vi "fun_TimeLength2Points(ClusterOfSweepPara).vi"(10 "HDAWG Sample Rate (2.4GSa/s)":dbl=2400000000.0 format="%#_13p", 11 "AWG Sweep Parameters Time length (s)":cluster{"End":dbl, "Step":dbl, "Start":dbl}={"End"=1.5e-05, "Step"=2.0833e-08, "Start"=2e-07} caption="Sweep Parameters" {"End" min=0.0 max=40000.0 step=1.0 format="%#.3ps"; "Step" format="%.3ps"; "Start" min=0.0 max=12000000000.0 step=100000000.0 format="%#.3ps"}) -> (3 "AWG Points":cluster{"End":dbl, "Step":dbl, "Start":dbl} caption="Points" {"End" min=0.0 max=40000.0 step=1.0; "Start" min=0.0 max=12000000000.0 step=100000000.0})   [LabVIEW 2016]
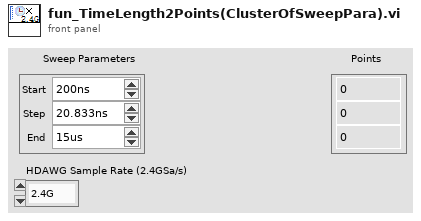
[diagram p1: front panel]
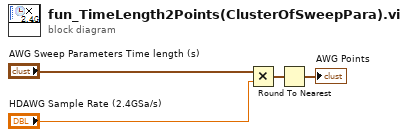
[diagram p0: block diagram]
diagram:
  n1 = Multiply(x="AWG Sweep Parameters Time length (s)", y="HDAWG Sample Rate (2.4GSa/s)") -> (x*y=w4:cluster{"End":dbl, "Step":dbl, "Start":dbl})
  n2 = Round To Nearest(number=w4) -> (nearest integer value=→"AWG Points":cluster{"End":dbl, "Step":dbl, "Start":dbl})
